vi "CAN-viewer-MPS(10).vi"() -> ()   [LabVIEW 2010]
uses:
  <vilib>/nican/nican.llb/ncNetAttr.ctl
  <vilib>/Utility/miscctls.llb/LVRowAndColumnUnsignedTypeDef.ctl
panel:
  out "Wheel RPM":dbl(knob) scale=0.0..1400.0
  out "Headlights":bool
  in  "Interface":string(combo)="CAN0"
  in  "stop":bool
  in  "Baudrate":u32=500000
  out "Motor Current (mA)":dbl
  in  "ID filter(hex)":u32 format="%.0x"
  out "Output Array 1":string[][](table)
  in  "Filter":bool
  # "CAN Messages"
  # "CAN Messages"
  # "RECEIVING MODE"
  # "This VI should be used to read CAN messages.\n\nThe section to the left has been created for you to display data received.\n\nThe section at the bottom should be implemented when using the RC car to gain full functionality.\n\n\nUse this button to stop the VI."
  # "Car Dashboard"
  # "STATUS REPLIES"
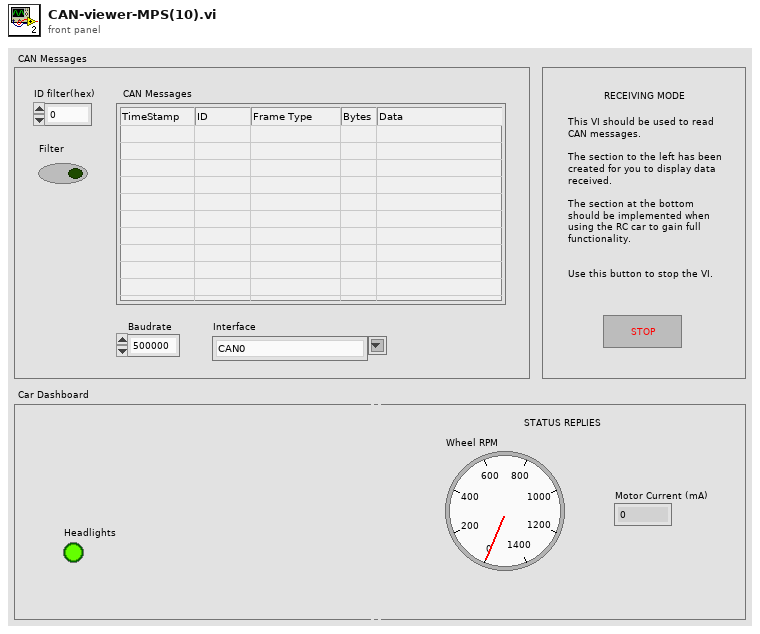
[diagram p1: front panel]
types:
  T1 = typedef "LVRowAndColumnUnsignedTypeDef.ctl" = cluster{"Row":u32, "Column":u32}
  T2 = typedef "ncNetAttr.ctl" = cluster{"Start On Open":enum32{"FALSE", "TRUE"}, "Baud Rate":u32, "Read Queue Length":u32, "Write Queue Length":u32, "Standard Comparator":u32, "Standard Mask":u32, "Extended Comparator":u32, "Extended Mask":u32}
  T3 = typedef "xobjhandle.ctl" = u32
  T4 = typedef "CanFrameTimed.ctl" = cluster{"Timestamp":dbl, "ArbitrationId":u32, "IsRemote":u8, "DataLength":u8, "Data":u8[]}
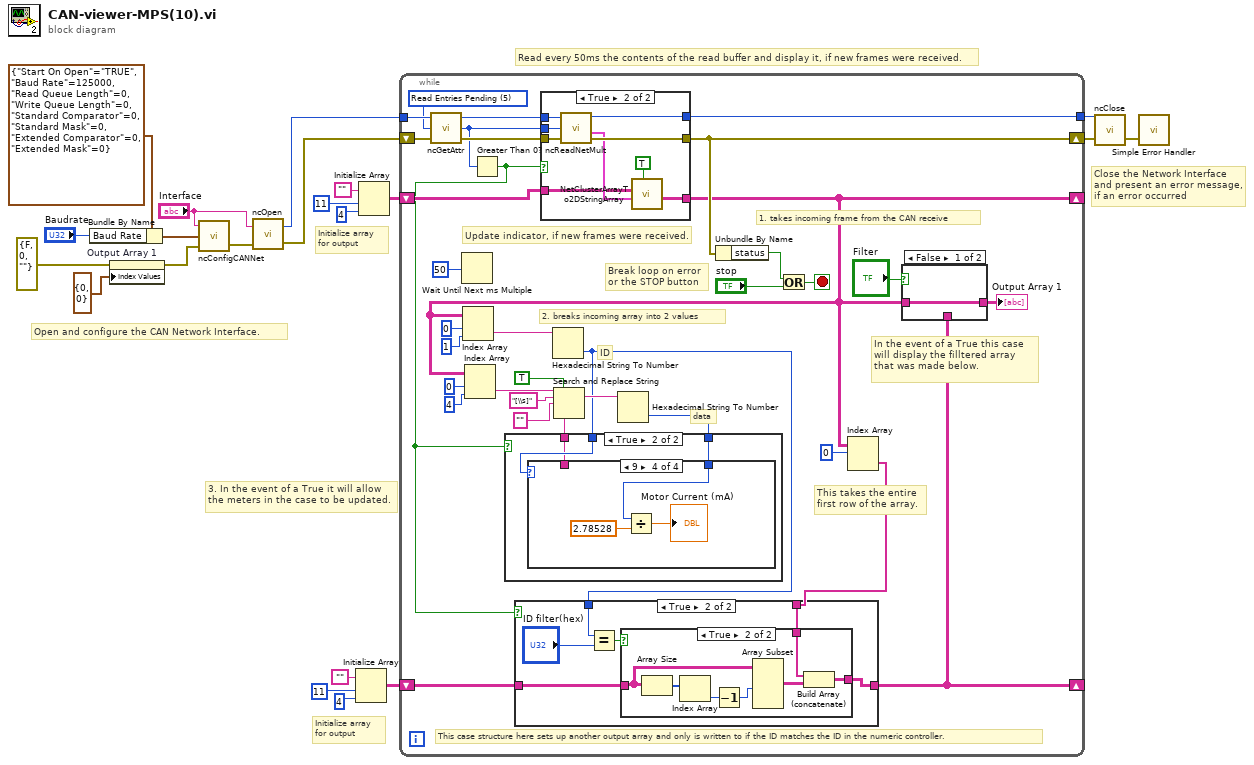
[diagram p0: block diagram]
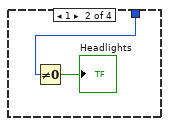
[diagram p7: hidden frame]
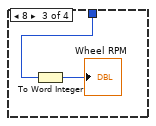
[diagram p8: hidden frame]
diagram:
  # "3. In the event of a True it will allow the meters in the case to be updated."
  # "Initialize array \nfor output"
  # "Initialize array \nfor output"
  # "Close the Network Interface \nand present an error message, \nif an error occurred"
  # "Read every 50ms the contents of the read buffer and display it, if new frames were received."
  # "Open and configure the CAN Network Interface."
  n1 = Bundle By Name(cluster=T2 {"Start On Open"=enum."TRUE", "Baud Rate"=125000, "Read Queue Length"=0, "Write Queue Length"=0, "Standard Comparator"=0, "Standard Mask"=0, "Extended Comparator"=0, "Extended Mask"=0} ("CAN Network Interface Config"), "Baud Rate"="Baudrate") -> (w19:T2)
  n2 = property on="Output Array 1" class="Tbl (strict)"(error in=errorcluster {"status"=FALSE, "code"=0, "source"=""} ("Error in"), "Index Values"=T1 {"Row"=0, "Column"=0}) -> (error out=w1:errorcluster)  [unwired: 1 in, 1 out]
  n3 = call <vilib>:"ncConfigCANNet.vi"("Error in"=w1, "CAN Network Interface Config"=w19, "ObjName"="Interface") -> ("Error out"=w17:errorcluster)  [unwired: 2 out]
  n4 = call <vilib>:"ncOpen.vi"("Error in"=w17, "ObjName"="Interface") -> ("Error out"=w15:errorcluster, "ObjHandle out"=w16:T3)
  n5 = Initialize Array("", 11 ("Dimension Size"), 4 ("Dimension Size")) -> (w4:string[][])
  n6 = Initialize Array("", 11 ("Dimension Size"), 4 ("Dimension Size")) -> (w10:string[][])
  n7 = while {
    shift-left: w10 -> [w49]
    shift-right: [w22] -> _
    tunnel: [w50] -> w12
    tunnel: w16 -> [w48]
    shift-left: w15 -> [w47]
    shift-right: [w52] -> w14
    shift-right: [w33] -> _
    shift-left: w4 -> [w38]
    stop <- w51 stop-if-true
    w44 = u32 5 items=["(reserved)", "Protocol Version", "Software Version", "Object State", "(reserved)", "Read Entries Pending", "Write Entries Pending", "ReadMult Size for Notification", "Listen Only?", "Self Reception?", "Transmit Error Counter", "Receive Error Counter", "Single Shot Transmit?", "Series 2 Filter Mode", "Series 2 Mask", "Series 2 Comparator", "Serial Number", "Form Factor", "Series", "Transceiver Type", "Interface Number", "Series 2 Error/Arb Capture", "Transceiver Mode", "Transceiver External Outputs", "Transceiver External Inputs", "Start Trigger Behavior", "Log Comm Warnings", "User RTSI Frame", "Transmit Mode", "Log Start Trigger?", "Timestamp Format", "Master Timebase Rate", "Virtual Bus Timing"] ("AttrId")
    # "Break loop on error or the STOP button"
    # "In the event of a True this case will display the filltered array that was made below."
    # "This takes the entire first row of the array."
    # "This case structure here sets up another output array and only is written to if the ID matches the ID in the numeric controller."
    # "data"
    # "ID"
    # "2. breaks incoming array into 2 values"
    # "1. takes incoming frame from the CAN receive"
    # "Update indicator, if new frames were received."
    n8 = call <vilib>:"ncGetAttr.vi"("Error in"=w47, "AttrId"=w44, "ObjHandle in"=w48) -> ("Error out"=w46:errorcluster, "AttrValue"=w24:u32, "ObjHandle out"=w45:T3)
    n9 = Wait Until Next ms Multiple(millisecond multiple=u32 50) -> ()  [unwired: 1 out]
    n10 = Greater Than 0?(x=w24) -> (x > 0?=w25:bool)
    n11 = case shown="True" w25 {
      tunnel: [w83 w93] -> w52
      tunnel: [w84 w91] -> w50
      tunnel: w49 -> [w82 w90]
      tunnel: w24 -> [_ w89]
      tunnel: w46 -> [w83 w88]
      tunnel: w45 -> [w84 w87]
      tunnel: [w82 w85] -> w22
      frame False {
      }
      frame True {
        n12 = call <vilib>:"ncReadNetMult.vi"("ObjHandle in"=w87, "Requested Number of Frames"=w89, "Error in"=w88) -> ("ObjHandle out"=w91:T3, "Data"=w92:T4[], "Error out"=w93:errorcluster)  [unwired: 1 out]
        n13 = call <vilib>:"NetClusterArrayTo2DStringArray.vi"("Hexadecimal?"=TRUE, "Data from ncReadNetMult"=w92, "Input Array"=w90) -> ("Output Array"=w85:string[][])  [unwired: 8 out]
      }
    }
    n14 = Index Array(array=w22, index (row)=0 ("Dimension Size"), index (col)=1 ("Dimension Size")) -> (element=w41:string)
    n15 = Index Array(array=w22, index (row)=0 ("Dimension Size"), index (col)=4 ("Dimension Size")) -> (element=w31:string)
    n16 = Hexadecimal String To Number(string=w41) -> (number=w23:u32)  [unwired: 3 out]
    n17 = Search and Replace String(replace all?=TRUE ("replace all? (F)"), input string=w31, search string="[\\s]", replace string="" ("replace string (\"\")")) -> (result string=w28:string)  [unwired: 4 in, 3 out]
    n18 = Hexadecimal String To Number(string=w28) -> (number=w32:u32)  [unwired: 3 out]
    n19 = case shown="True" w25 {
      tunnel: w23 -> [_ w74]
      tunnel: w32 -> [_ w73]
      tunnel: w28 -> [_ w72]
      frame False {
      }
      frame True {
        n20 = case shown="9" w74 {
          tunnel: w73 -> [_ w75 w78 w80]
          tunnel: w72 -> [_ _ _ _]
          frame 0, Default {
          }
          frame 1 {
            n21 = Not Equal To 0?(x=w75) -> (x != 0?=→"Headlights":bool)
          }
          frame 8 {
            n22 = To Word Integer(number=w78) -> (16bit integer=→"Wheel RPM":i16)
          }
          frame 9 {
            n23 = Divide(x=w80, y=2.78528) -> (x/y=→"Motor Current (mA)":dbl)
          }
        }
      }
    }
    n24 = Unbundle By Name(w52) -> ("status"=w53:bool)
    n25 = Or(x=w53, y="stop") -> (x .or. y?=w51:bool)
    n26 = Index Array(array=w22, index (row)=0) -> (element=w36:string[])  [unwired: 1 in]
    n27 = case shown="True" w25 {
      tunnel: w23 -> [_ w62]
      tunnel: [w57 w58] -> w33
      tunnel: w38 -> [w57 w60]
      tunnel: w36 -> [_ w59]
      frame False {
      }
      frame True {
        n28 = Equal?(x=w62, y="ID filter(hex)") -> (x = y?=w61:bool)
        n29 = case shown="True" w61 {
          tunnel: [w64 w67] -> w58
          tunnel: w59 -> [_ w66]
          tunnel: w60 -> [w64 w65]
          frame False {
          }
          frame True {
            n30 = Array Size(array=w65) -> (size(s)=w70:i32[])
            n31 = Index Array(array=w70) -> (element=w69:i32)  [unwired: 1 in]
            n32 = Decrement(x=w69) -> (x-1=w68:i32)
            n33 = Array Subset(array=w65, length (row)=w68) -> (w71:string[][])  [unwired: 3 in]
            n34 = Build Array (concatenate)(w66, w71) -> (w67:string[][])
          }
        }
      }
    }
    n35 = case shown="False" "Filter" {
      tunnel: w22 -> [w55 _]
      tunnel: w33 -> [_ w56]
      tunnel: [w55 w56] -> w35
      frame False {
      }
      frame True {
      }
    }
    "Output Array 1" <- w35
  }
  n36 = call <vilib>:"ncClose.vi"("Error in"=w14, "ObjHandle in"=w12) -> ("Error out"=w13:errorcluster)  [unwired: 1 out]
  n37 = call <vilib>:"Simple Error Handler.vi"("error in (no error)"=w13) -> ()  [unwired: 1 in, 8 out]
